vi "Create Shared Resources.vi"(8 "error in":errorcluster, 10 "custom device ref":T1=18446744073709551615 format="%.0x", 11 "shared resources factory in":refnum<class "Shared Resources Factory.lvclass">) -> (0 "error out":errorcluster, 2 "shared resources":refnum<class "Shared Resources.lvclass">, 3 "shared resources factory out":refnum<class "Shared Resources Factory.lvclass">)   [LabVIEW 2020, in "Communication Bus Template Engine.lvlib" / "Interfaces.lvlib" / "Shared Resources Factory.lvclass"]
uses:
  Shared Resources Factory.lvclass
  <vilib>/NI VeriStand/Custom Device API/Custom Device Item Ref.ctl
  Shared Resources/Shared Resources.lvclass
  <vilib>/NI VeriStand/Custom Device API/Custom Device API.lvlib
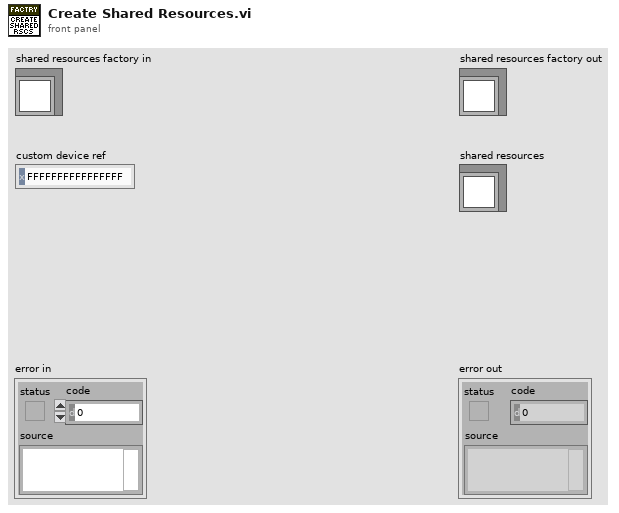
[diagram p1: front panel]
types:
  T1 = typedef "Custom Device API.lvlib/Custom Device Item Ref.ctl" = u64
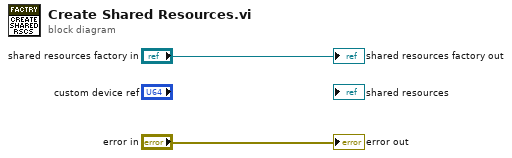
[diagram p0: block diagram]
diagram:
  "error out" <- "error in"
  "shared resources factory out" <- "shared resources factory in"
